vi "Find Node Attribute from File Recursively.vi"(7 "XPath":T5=enum."@Name", 8 "error in":errorcluster, 9 "Parent":string[](array[string]), 10 "Path to XML document":path caption="Path to Item XML Document", 11 "VI Data":T1[](array[typedef])) -> (0 "error out":errorcluster, 3 "VI Data out":T1[](array[typedef]))   [LabVIEW 2020, in "VI Properties Editor.lvlib"]
uses:
  VI Properties Editor.lvlib
  <vilib>/xml/NI_XML.lvlib
  CTLs/XPath Get Attribute.ctl
  <vilib>/xml/Load XML String.vi
  <vilib>/xml/Close Reference(Node).vi
  <vilib>/picture/picture.llb/imagedata.ctl
  CTLs/VI Properties.ctl
  CTLs/Control Properties.ctl
  CTLs/VI Data.ctl
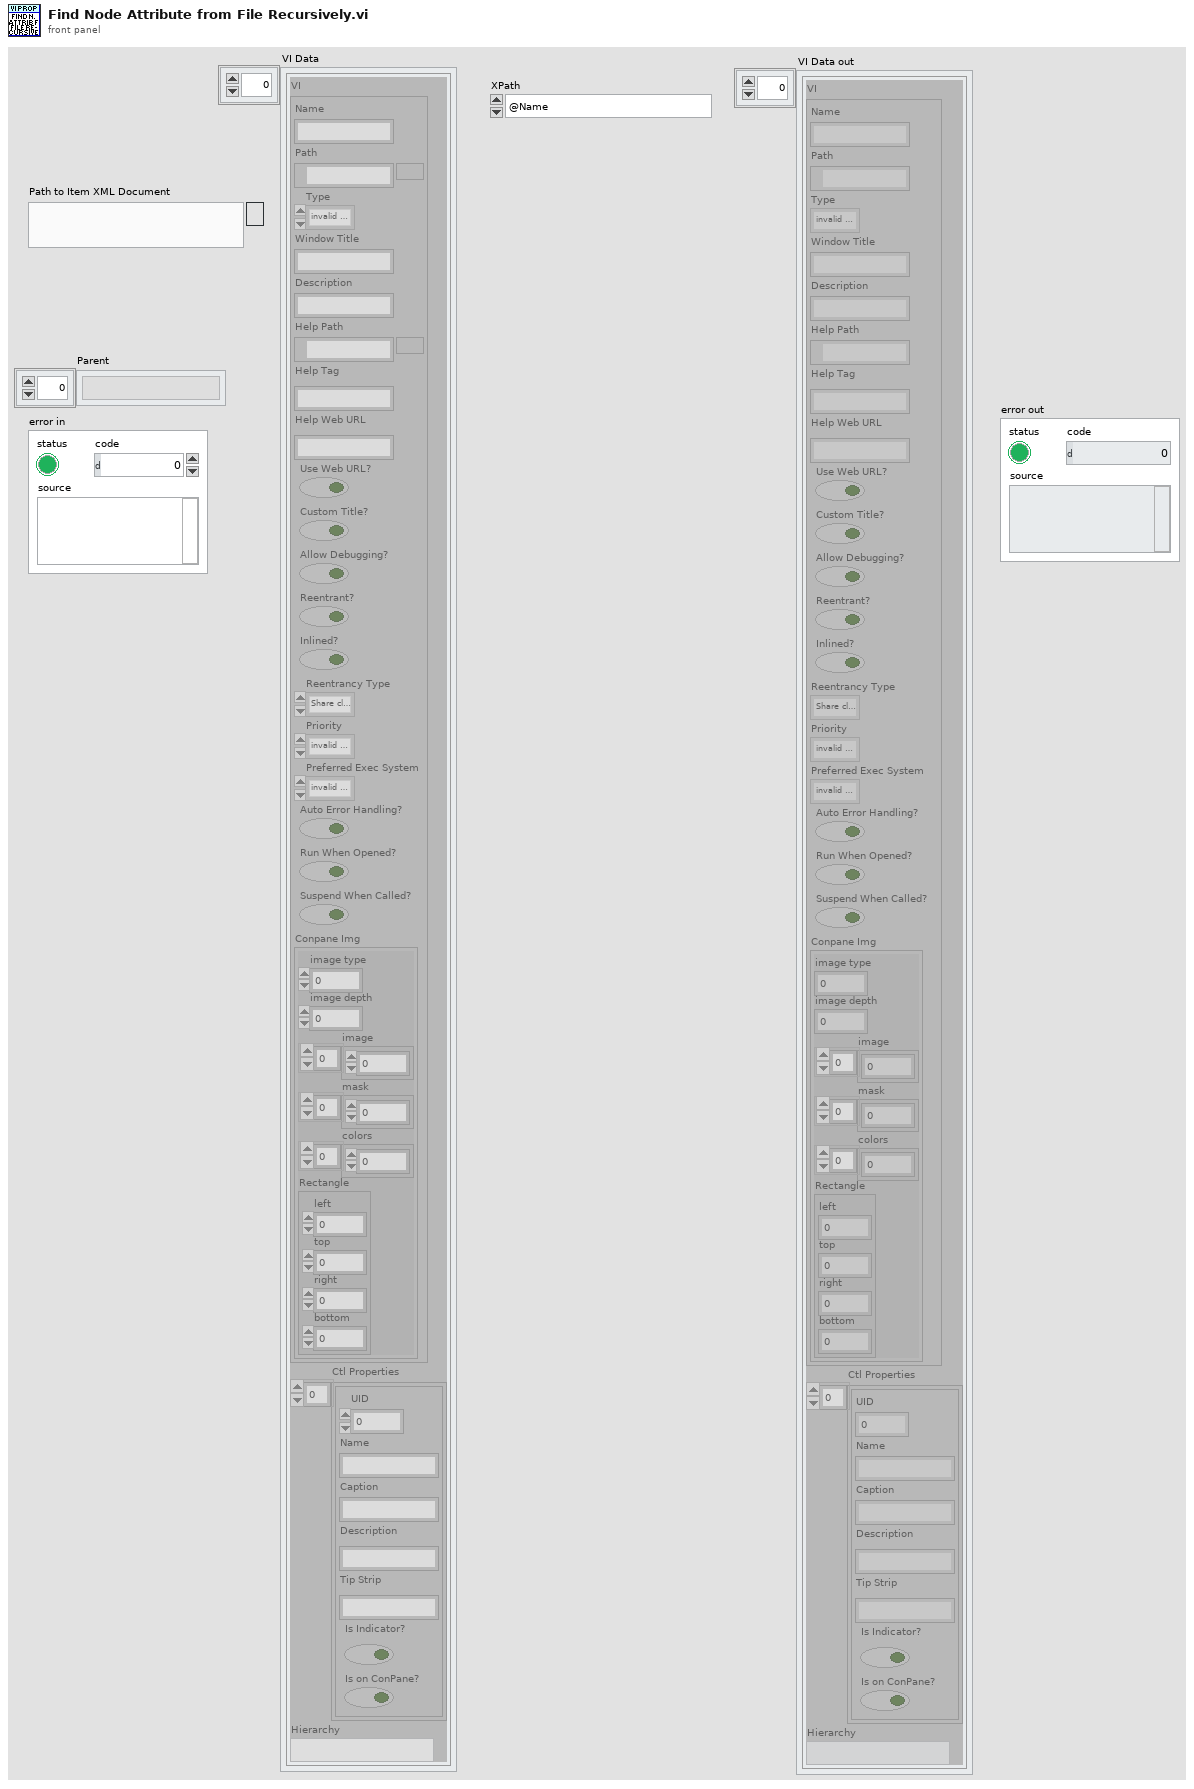
[diagram p1: front panel]
types:
  T1 = typedef "VI Properties Editor.lvlib/VI Data.ctl" = cluster{"VI":T2, "Ctl Properties":T4[], "Hierarchy":string}
  T2 = typedef "VI Properties Editor.lvlib/VI Properties.ctl" = cluster{"Name":string, "Path":path, "Type":enum32{"invalid VI type", "Standard VI", "Control VI", "Global VI", "Polymorphic VI", "Configuration VI", "SubSystem", "Facade VI", "Method VI", "Statechart Diagram VI"}, "Window Title":string, "Description":string, "Help Path":path, "Help Tag":string, "Help Web URL":string, "Use Web URL?":bool, "Custom Title?":bool, "Allow Debugging?":bool, "Reentrant?":bool, "Inlined?":bool, "Reentrancy Type":enum16{"Share clones between instances", "Preallocate clone for each instance"}, "Priority":enum32{"invalid priority", "background priority", "normal priority", "above normal priority", "high priority", "time critical priority", "subroutine"}, "Preferred Exec System":enum32{"invalid execution system", "user interface", "standard", "instrument i/o", "data acquisition", "other 1", "other 2", "same as caller"}, "Auto Error Handling?":bool, "Run When Opened?":bool, "Suspend When Called?":bool, "Conpane Img":T3}
  T3 = typedef "imagedata.ctl" = cluster{"image type":i32, "image depth":i32, "image":u8[], "mask":u8[], "colors":u32[], "Rectangle":cluster{"left":i16, "top":i16, "right":i16, "bottom":i16}}
  T4 = typedef "VI Properties Editor.lvlib/Control Properties.ctl" = cluster{"UID":i32, "Name":string, "Caption":string, "Description":string, "Tip Strip":string, "Is Indicator?":bool, "Is on ConPane?":bool}
  T5 = typedef "VI Properties Editor.lvlib/XPath Get Attribute.ctl" = enum16{"Item[@Type='VI']/@URL", "Item[@Type='LVClass']/@URL", "Item[@Type='Library']/@URL", "Item[@Type='Folder' and not (@URL)]/@Name", "@Name"}
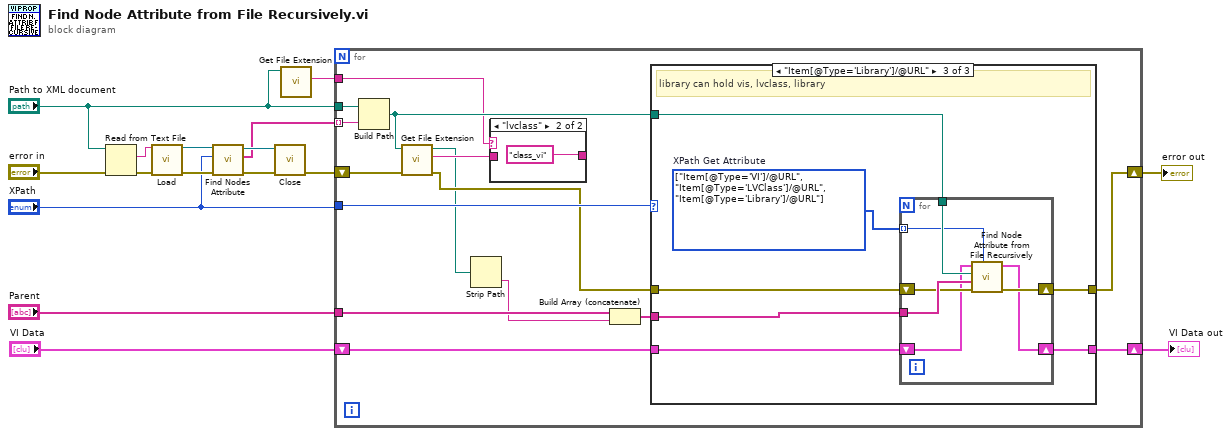
[diagram p0: block diagram]
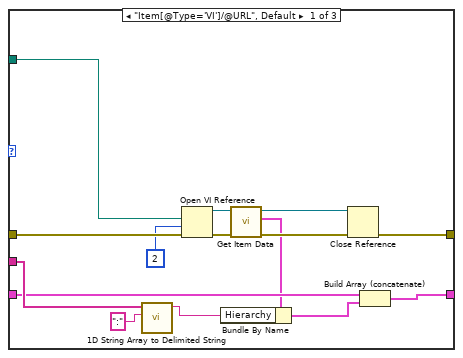
[diagram p3: hidden frame]
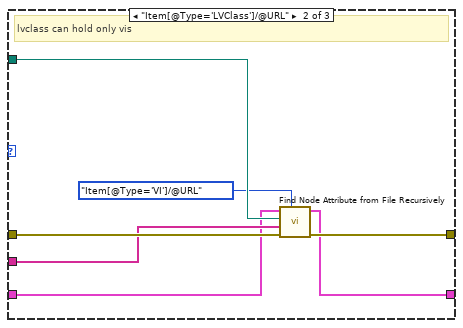
[diagram p4: hidden frame]
diagram:
  n1 = Read from Text File(file (use dialog)="Path to XML document", error in="error in") -> (text=w12:string, error out=w13:errorcluster)  [unwired: 2 in, 2 out]
  n2 = call-poly <vilib>:"Load.vi"("XML string"=w12, "error in (no error)"=w13) -> ("DOM document out"=w9:refnum<k20>, "error out"=w11:errorcluster)  [unwired: 11 in, 1 out]
  n3 = call "Find Nodes Attribute.vi"("error in"=w11, "XPath"="XPath", "Node in"=w9) -> ("error out"=w8:errorcluster, "Attribute"=w1:string[], "Node out"=w2:refnum<k20>)  [unwired: 6 in]
  n4 = call-poly <vilib>:"Close.vi"("error in (no error)"=w8, "node"=w2) -> ("error out"=w10:errorcluster)  [unwired: 7 in]
  n5 = call <vilib>:"Get File Extension.vi"("file"="Path to XML document") -> ("lowercase file extension"=w6:string)  [unwired: 6 in, 4 out]
  n6 = for {
    shift-right: [w31] -> w15
    shift-left: w10 -> [w26]
    tunnel: "XPath" -> [w27]
    tunnel: "Parent" -> [w30]
    tunnel: "Path to XML document" -> [w29]
    tunnel: w1 -> [w28] mode=indexing
    tunnel: w6 -> [w22]
    shift-right: [w18] -> w3
    shift-left: "VI Data" -> [w19]
    n7 = Build Path(base path=w29, name or relative path=w28) -> (appended path=w25:path)
    n8 = call <vilib>:"Get File Extension.vi"("error in (no error)"=w26, "file"=w25) -> ("error out"=w24:errorcluster, "lowercase file extension"=w23:string, "dup file"=w17:path)  [unwired: 5 in, 2 out]
    n9 = Strip Path(path=w17) -> (name=w20:string)  [unwired: 1 out]
    n10 = case shown="\"lvclass\"" w22 {
      tunnel: w23 -> [w32 _]
      tunnel: [w32 "class_vi"] -> _
      frame Default {
      }
      frame "lvclass" {
      }
    }
    n11 = Build Array (concatenate)(w30, w20) -> (w21:string[])
    n12 = case shown="\"Item[@Type='Library']/@URL\"" w27 {
      tunnel: [w45 w55 w62] -> w31
      tunnel: w21 -> [w40 w51 w61]
      tunnel: w24 -> [w48 w54 w60]
      tunnel: w25 -> [w38 w53 w59]
      tunnel: w19 -> [w37 w50 w57]
      tunnel: [w41 w49 w56] -> w18
      frame "Item[@Type='VI']/@URL", Default {
        n13 = call <vilib>:"1D String Array to Delimited String.vi"("delimiter"=":", "string array"=w40) -> ("delimited string"=w35:string)  [unwired: 9 in]
        n14 = Open VI Reference(vi path=w38, options=2, error in (no error)=w48) -> (vi reference=w43:refnum<vi>, error out=w47:errorcluster)  [unwired: 3 in]
        n15 = call "Get Item Data.vi"("error in (no error)"=w47, "VI Ref"=w43) -> ("error out"=w44:errorcluster, "VI Data"=w36:T1, "VI Ref out"=w42:refnum<vi>)  [unwired: 7 in]
        n16 = Bundle By Name(cluster=w36, "Hierarchy"=w35) -> (w34:T1)
        n17 = Close Reference(reference=w42, error in (no error)=w44) -> (error out=w45:errorcluster)
        n18 = Build Array (concatenate)(w37, w34) -> (w41:T1[])
      }
      frame "Item[@Type='LVClass']/@URL" {
        # "lvclass can hold only vis"
        n19 = call "Find Node Attribute from File Recursively.vi"("XPath"=XPath_Get_Attribute."Item[@Type='VI']/@URL", "error in"=w54, "Parent"=w51, "Path to XML document"=w53, "VI Data"=w50) -> ("error out"=w55:errorcluster, "VI Data out"=w49:T1[])  [unwired: 5 in]
      }
      frame "Item[@Type='Library']/@URL" {
        w58 = T5[] [enum."Item[@Type='VI']/@URL", enum."Item[@Type='LVClass']/@URL", enum."Item[@Type='Library']/@URL"] items=["Item[@Type='VI']/@URL", "Item[@Type='LVClass']/@URL", "Item[@Type='Library']/@URL", "Item[@Type='Folder' and not (@URL)]/@Name", "@Name"]  # XPath Get Attribute
        # "library can hold vis, lvclass, library"
        n20 = for {
          tunnel: w61 -> [w68]
          tunnel: w59 -> [w66]
          shift-right: [w69] -> w62
          shift-left: w60 -> [w67]
          tunnel: w58 -> [w65] mode=indexing
          shift-right: [w63] -> w56
          shift-left: w57 -> [w64]
          n21 = call "Find Node Attribute from File Recursively.vi"("XPath"=w65, "error in"=w67, "Parent"=w68, "Path to XML document"=w66, "VI Data"=w64) -> ("error out"=w69:errorcluster, "VI Data out"=w63:T1[])  [unwired: 5 in]
        }
      }
    }
  }
  "error out" <- w15
  "VI Data out" <- w3
